vi "Get Keypad.vi"(8 "error in (no error)":errorcluster, 10 "Keypad Screen":dbl, 11 "ATM Controller in":refnum<class "ATM Controller.lvclass">) -> (0 "error out":errorcluster, 3 "ATM Controller out":refnum<class "ATM Controller.lvclass">)   [LabVIEW 2019, in "ATM Controller.lvlib" / "ATM Controller.lvclass"]
uses:
  ATM Controller.lvclass
  ATM Controller.lvclass/ATM Controller.ctl
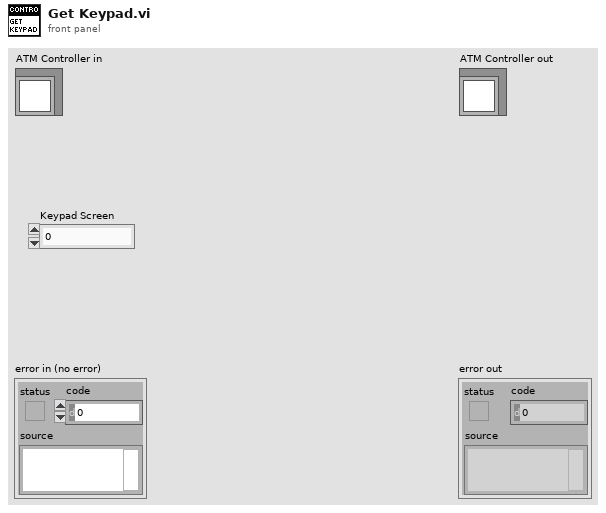
[diagram p1: front panel]
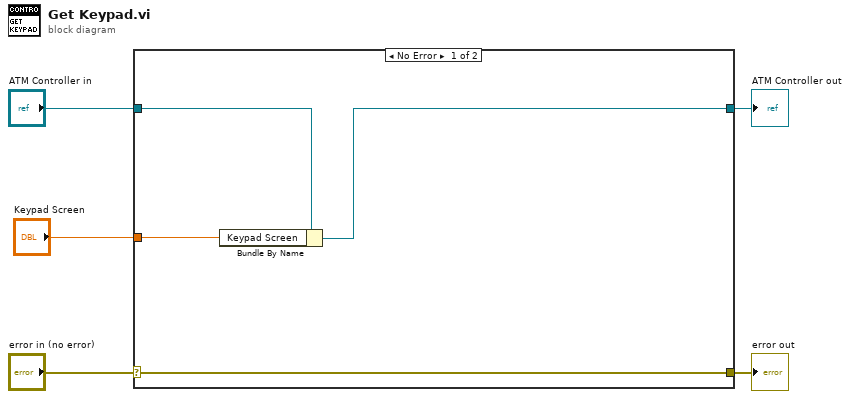
[diagram p0: block diagram]
diagram:
  n1 = case shown="No Error" "error in (no error)" {
    selector: "error in (no error)" -> [w9 w11]
    tunnel: [w9 w11] -> w4
    tunnel: [w6 w10] -> w2
    tunnel: "ATM Controller in" -> [w7 w10]
    tunnel: "Keypad Screen" -> [w8 _]
    frame No Error {
      n2 = Bundle By Name(cluster=w7, "Keypad Screen"=w8) -> (w6:refnum<class "ATM Controller.lvclass">)
    }
    frame Error {
    }
  }
  "error out" <- w4
  "ATM Controller out" <- w2
